vi "Streamlined FPGA--smooth window of 4.vi"() -> ()   [LabVIEW 2009]
uses:
  <vilib>/eio/EIONode/EIONode.xnode
  <vilib>/rvi/eio/nirviEIOImplementation/nirviEIOImplementation.xnode
  <vilib>/rvi/eio/common/nirviEmuTemplateMethod_noerrors.vi
  <vilib>/rvi/eio/common/nirviEmuClasses.ctl
  Instance           3 24Saved   Streamlined FPGA .vi
  Instance           4 24Saved   Streamlined FPGA .vi
  Instance           5 24Saved   Streamlined FPGA .vi
  Instance           2 24Saved   Streamlined FPGA .vi
  <vilib>/rvi/DataTransferAndStorage/Container/XNode/niFpgaContainer.xnode
  <vilib>/rvi/interface/RandomDataEmulation/niFpgaRandomDataHandleErrors.vi
  <vilib>/rvi/interface/RandomDataEmulation/nirviRandomDataFPGAFIFO.vi
  <vilib>/rvi/DataTransferAndStorage/Container/Common/niFpgaContainerMethod.ctl
  <vilib>/rvi/DataTransferAndStorage/Container/Common/niFpgaTransferTypeControl.ctl
panel:
  in  "smooth":bool
  out ">= x":bool
  out ">= y":bool
  out "xmax":i32
  out "xval":i32
  out "xmin":i32
  out ">=":bool
  in  "Rec2 Ymin":i32
  in  "Rec2 Xmin":i32
  in  "Rec1 Ymin":i32
  in  "Rec1 Xmin":i32
  in  "Rec2 Ymax":i32
  in  "Rec1 Ymax":i32
  in  "Rec2 Xmax":i32
  in  "Rec1 Xmax":i32
  out "sort!":bool
  in  "Maximum Width":i16
  in  "Maximum Height":i16
  in  "trigger on all":bool
  out "sort pulse":i16
  in  "Baselines":i16[](array[numeric])=[0, 0, 0, 0]
  in  "Sb":i8(ring)=1 items=["PMT1", "PMT2", "PMT3", "PMT4"]
  in  "Sa":i8(ring) items=["PMT1", "PMT2", "PMT3", "PMT4"]
  in  "Sort Case":i8(ring)=1 items=["FP", "Magnitude"]
  out "Full 2":bool
  in  "sort?":bool
  out "Drop counter":u32
  out "sort counter":u32
  in  "PMT to detect drops on":u8
  in  "Minimum Height":i16
  in  "Minimum Width":i16
  in  "Ticks between acquires (Ticks)":u32=200
  in  "Gain 1":i16(slide) scale=-32767.0..32767.0
  in  "Gain 2":i16(slide) scale=-32767.0..32767.0
  in  "Gain 3":i16(slide) scale=-32767.0..32767.0
  in  "Gain 4":i16(slide) scale=-32767.0..32767.0
  in  "amplitude":i16
  in  "1/Frequency \n(ticks)":u32
  in  "Burst \nCycles":i32
  in  "delay [us]":u32=20 min=1 max=8000
  # "Acquisition and Detection"
  # "FP and Sorting Parameters"
  # "Sorting Pulse\nGenerator"
  # "Events"
  # "PMT Controls"
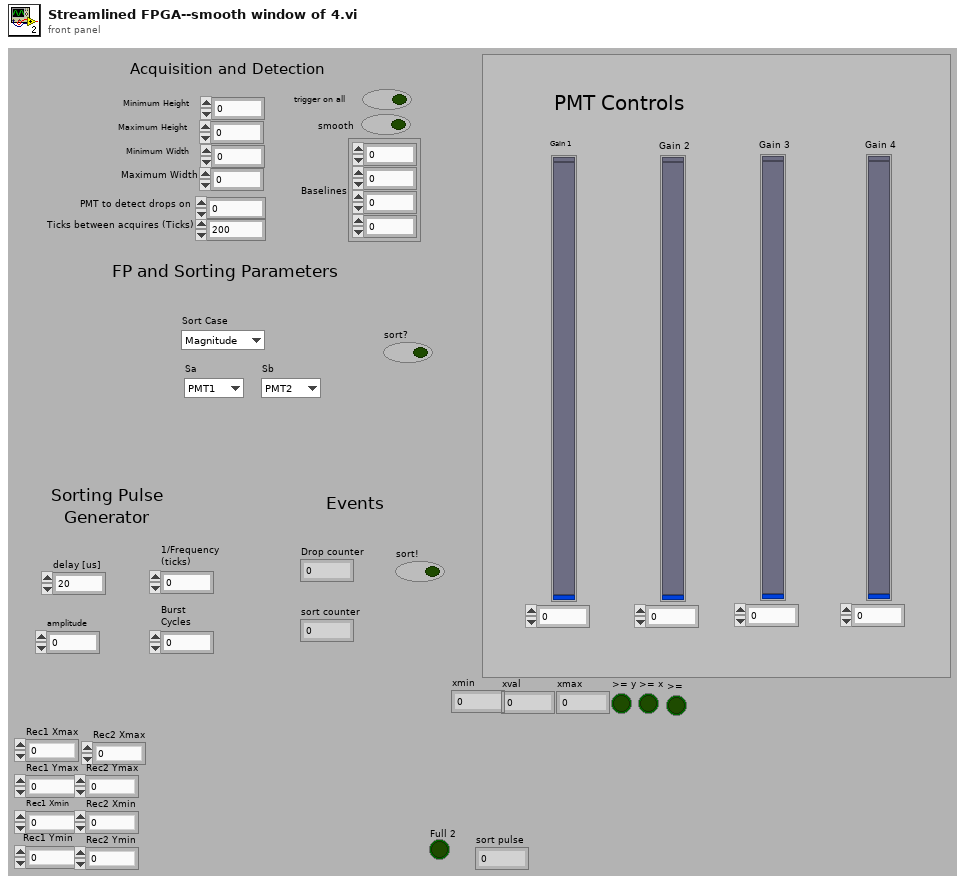
[diagram p1: front panel]
types:
  T1 = typedef "nirviEmuClasses.ctl" = enum16{"IO Read", "IO Write", "Method", "Property Read", "Property Write"}
  T2 = typedef "niFpgaContainerMethod.ctl" = enum16{"Write", "Read", "Clear", "Get Number of Elements to Write", "Get Number of Elements to Read", "Enable", "Disable", "Flush and Disable", "Get Stream State"}
  T3 = typedef "niFpgaTransferTypeControl.ctl" = enum16{"Target-Scoped", "Host to Target - DMA", "Target to Host - DMA", "Peer to Peer Reader", "Peer to Peer Writer", "Bidirectional"}
  T4 = cluster{"Rec1 Xmax":i32, "Rec1 Ymax":i32, "Rec1 Xmin":i32, "Rec1 Ymin":i32, "Rec2 Xmax":i32, "Rec2 Ymax":i32, "Rec2 Xmin":i32, "Rec2 Ymin":i32}
  T5 = cluster{bool, "max":i16[], "sum":i32[], "time inside":i32, "time outside":i32, "timeoutside-1":i32}
  T6 = cluster{"maxes":i16[], "sums":i32[], "time inside":i32, "time outside":i32}
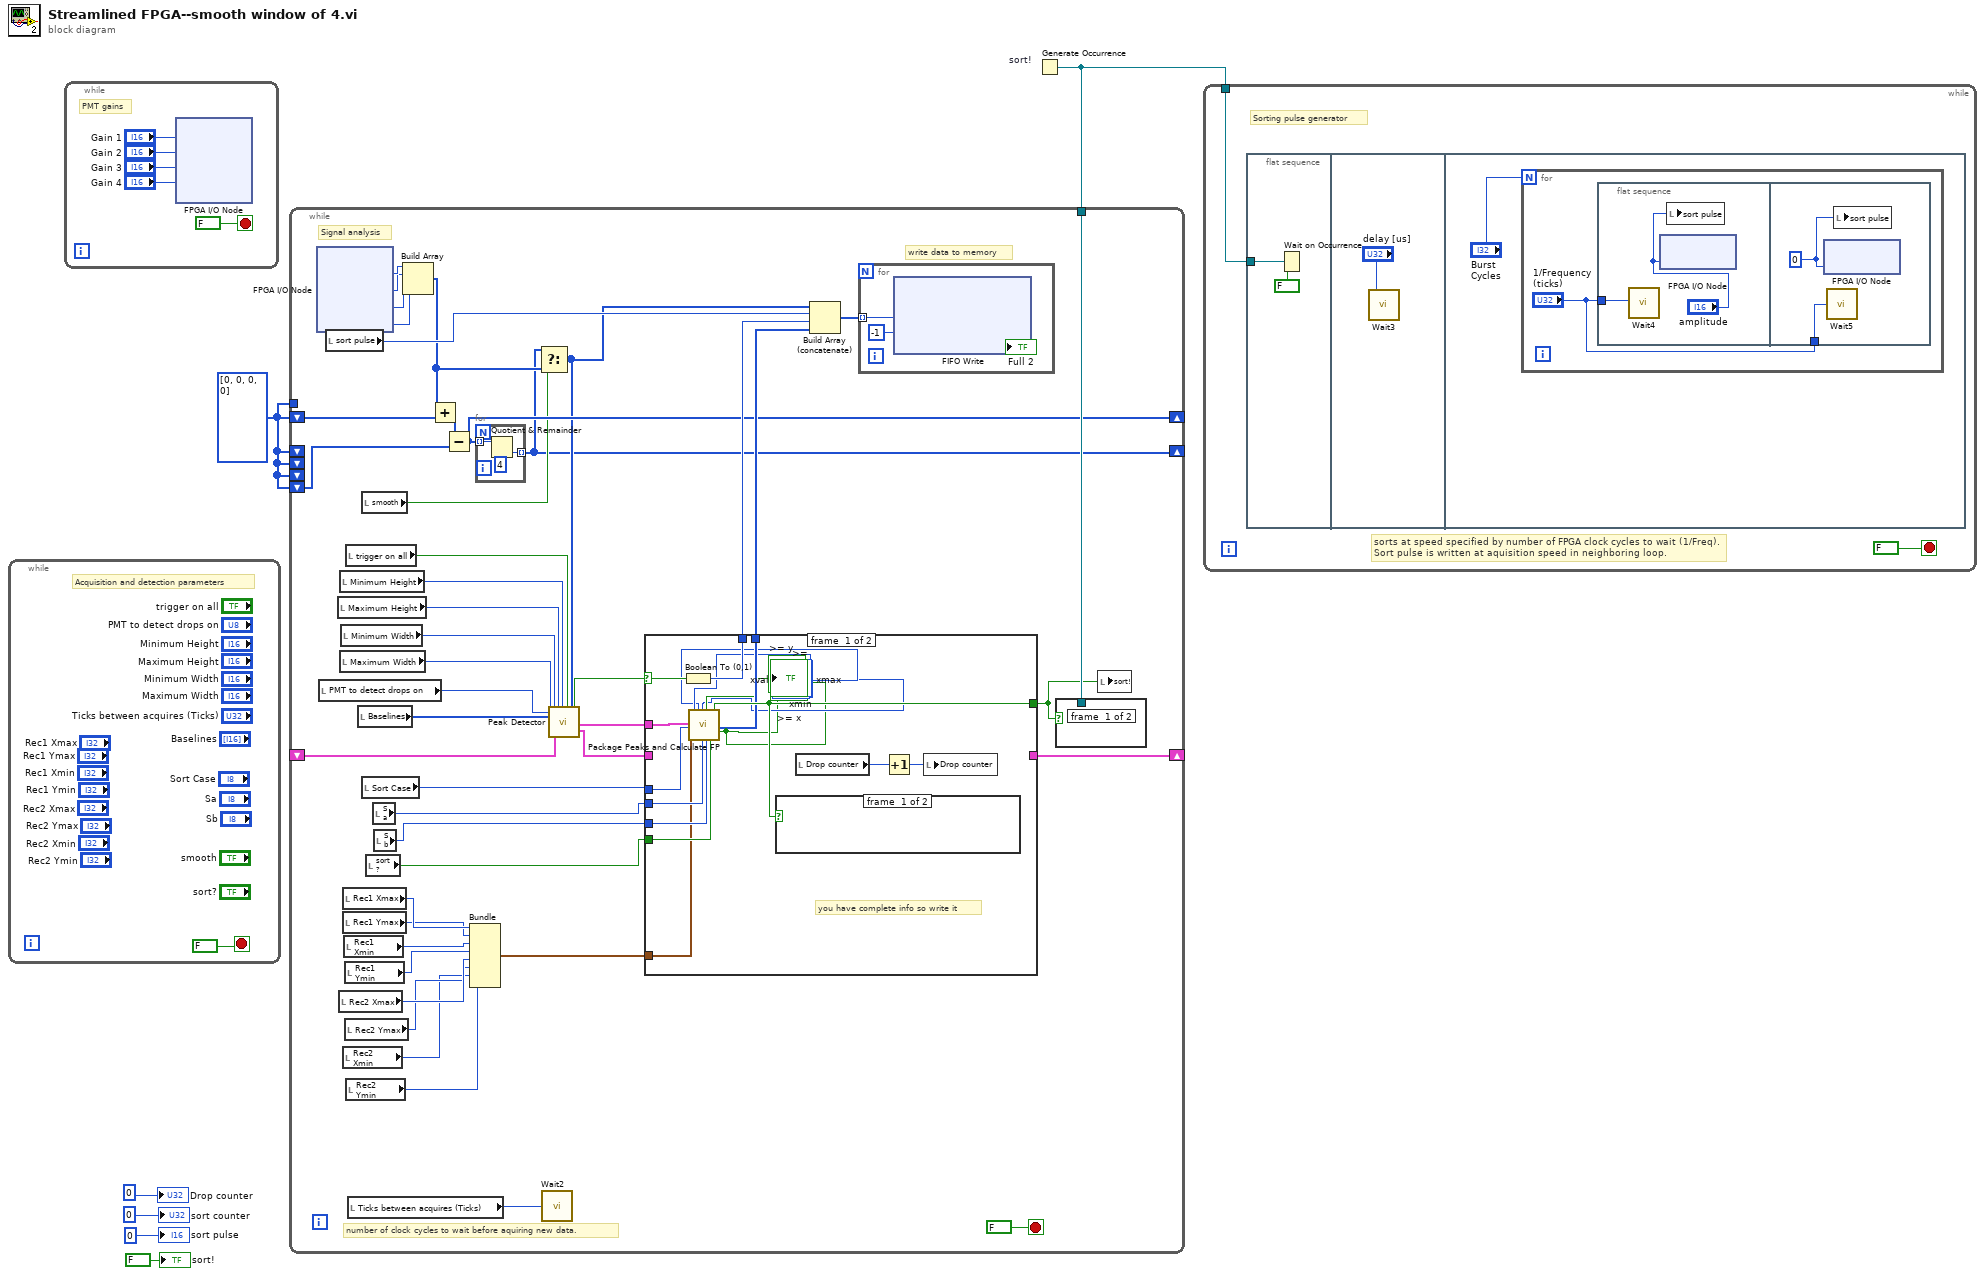
[diagram p0: block diagram]
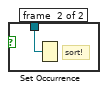
[diagram p2: hidden frame]
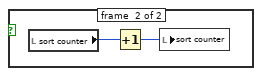
[diagram p3: hidden frame]
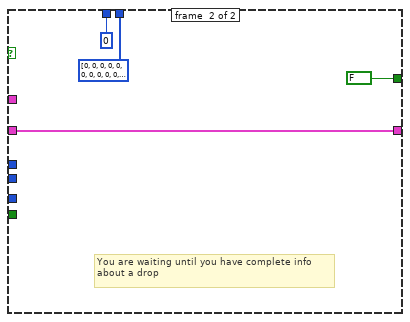
[diagram p4: hidden frame]
diagram:
  w1 = i32[] [0, 0, 0, 0] ("appended array")
  n1 = while {
    stop <- FALSE stop-if-true
    # "Acquisition and detection parameters"
  }
  n2 = while {
    stop <- FALSE stop-if-true
    # "PMT gains"
    n3 = xnode "FPGA I/O Node"("AO0"="Gain 1", "AO1"="Gain 2", "AO2"="Gain 3", "AO3"="Gain 4") -> ()  [unwired: 4 in, 4 out]
  }
  n4 = Generate Occurrence "sort!"() -> (w6:refnum<k4>)
  n5 = while {
    shift-right: [w100] -> _
    shift-left: _ -> [w87]
    tunnel: w6 -> [w85]
    shift-right: [w63] -> _
    shift-left: w1 -> [w64]
    shift-right: [w57] -> _
    shift-left: w1 -> [_]
    shift-left: w1 -> [_]
    shift-left: w1 -> [_]
    shift-left: w1 -> [w62]
    tunnel: w1 -> [_]
    stop <- FALSE stop-if-true
    # "number of clock cycles to wait before aquiring new data."
    # "Signal analysis"
    # "write data to memory"
    n6 = xnode "FPGA I/O Node"() -> ("AI0"=w99:i16, "AI1"=w98:i16, "AI2"=w97:i16, "AI3"=w96:i16)  [unwired: 4 in, 4 out]
    n7 = local read "PMT to detect drops on"() -> (w77:u8)
    n8 = local read "sort pulse"() -> (w84:i16)
    n9 = local read "Maximum Height"() -> (w80:i16)
    n10 = local read "Rec2 Xmax"() -> (w69:i32)
    n11 = local read "Minimum Height"() -> (w81:i16)
    n12 = local read "Maximum Width"() -> (w78:i16)
    n13 = local read "Minimum Width"() -> (w79:i16)
    n14 = local read "Rec1 Xmax"() -> (w73:i32)
    n15 = local read "Rec1 Ymax"() -> (w72:i32)
    n16 = local read "Rec2 Xmin"() -> (w67:i32)
    n17 = local read "Rec1 Xmin"() -> (w71:i32)
    n18 = local read "Rec1 Ymin"() -> (w70:i32)
    n19 = local read "Rec2 Ymax"() -> (w68:i32)
    n20 = local read "trigger on all"() -> (w86:bool)
    n21 = local read "Rec2 Ymin"() -> (w66:i32)
    n22 = local read "Ticks between acquires (Ticks)"() -> (w95:u32)
    n23 = local read "Baselines"() -> (w76:i16[])
    n24 = local read "smooth"() -> (w58:bool)
    n25 = local read "Sort Case"() -> (w94:i8)
    n26 = local read "sort?"() -> (w91:bool)
    n27 = local read "Sa"() -> (w93:i8)
    n28 = local read "Sb"() -> (w92:i8)
    n29 = Build Array(w99, w98, w97, w96) -> (w60:i16[])
    n30 = Add(x=w60, y=w64) -> (x+y=w61:i32[])
    n31 = Subtract(x=w61, y=w62) -> (x-y=w63:i32[])
    n32 = Bundle("Rec1 Xmax"=w73, "Rec1 Ymax"=w72, "Rec1 Xmin"=w71, "Rec1 Ymin"=w70, "Rec2 Xmax"=w69, "Rec2 Ymax"=w68, "Rec2 Xmin"=w67, "Rec2 Ymin"=w66) -> (w65:T4)  [unwired: 1 in]
    n33 = for {
      tunnel: [w103] -> w57 mode=indexing
      tunnel: w63 -> [w102] mode=indexing
      n34 = Quotient & Remainder(x=w102, y=4 ("AI3")) -> (floor(x/y)=w103:i32)  [unwired: 1 out]
    }
    n35 = Select(t=w57, s=w58, f=w60) -> (s? t:f=w59:i32[])
    n36 = call "Wait2"("Count(Ticks)"=w95) -> ()  [unwired: 1 out]
    n37 = call "Peak Detector.vi"("Maximum Width"=w78, "PMT to trigger on (0,1,2,3)"=w77, "Baselines"=w76, "Minimum Width"=w79, "shifts in"=w87, "Maximum Height"=w80, "Minimum Height"=w81, "trigger on all"=w86, "s1,s2,s3,s4"=w59) -> ("peak complete?"=w90:bool, "shifts out"=w88:T5, "peaks data"=w89:T6)  [unwired: 16 in]
    n38 = case shown="True" w90 {
      selector: w90 -> [w220 _]
      tunnel: [_ w231] -> w100
      tunnel: [w218 FALSE ("sort!")] -> w75
      tunnel: w94 -> [w216 _]
      tunnel: w93 -> [w224 _]
      tunnel: w92 -> [w223 _]
      tunnel: w91 -> [w222 _]
      tunnel: w88 -> [_ w231]
      tunnel: w89 -> [w221 _]
      tunnel: [w219 i16 0] -> w82
      tunnel: [w217 i32[] [0, 0, 0, 0, 0, 0, 0, 0, 0, 0, 0, 0] ("M1,M2,M3,M4,S1,S2,S3,S4,Tin,Tout,FP")] -> w74
      tunnel: w65 -> [w215 _]
      frame #0 {
        # "you have complete info so write it"
        n39 = Boolean To (0,1)(Boolean=w220) -> (0, 1=w219:i16)
        n40 = call "Package Peaks and Calculate FP.vi"("peaks data"=w221, "Sort Case"=w216, "Rectangle Positions"=w215, "Sa"=w224, "Sb"=w223, "sort?"=w222) -> ("xmin"=→"xmin":i32, "xval"=→"xval":i32, "xmax"=→"xmax":i32, ">="=→">=":bool, "sort!"=w218:bool, "M1,M2,M3,M4,S1,S2,S3,S4,Tin,Tout,FP,Sort?"=w217:i32[], ">= y"=→">= y" →">= x":bool)  [unwired: 14 in, 1 out]
        n41 = case shown="True" w218 {
          frame #0 {
          }
          frame #1 {
            n42 = local read "sort counter"() -> (w228:u32)
            n43 = Increment(x=w228) -> (x+1=w227:u32)
            n44 = local write "sort counter"(w227) -> ()
          }
        }
        n45 = local read "Drop counter"() -> (w226:u32)
        n46 = Increment(x=w226) -> (x+1=w225:u32)
        n47 = local write "Drop counter"(w225) -> ()
      }
      frame #1 {
        # "You are waiting until you have complete info about a drop"
      }
    }
    n48 = Build Array (concatenate)(w59, w84, w82, w74) -> (w83:i32[])
    n49 = for {
      tunnel: w83 -> [w108] mode=indexing
      n50 = xnode ("FIFO Write")("Element"=w108, "Timeout"=-1) -> ("Timed Out?"=→"Full 2":bool)  [unwired: 1 in, 1 out]
    }
    n51 = case shown="True" w75 {
      tunnel: w85 -> [_ w105]
      frame #0 {
      }
      frame #1 {
        # "sort!"
        n52 = Set Occurrence(w105) -> ()
      }
    }
    n53 = local write "sort!"(w75) -> ()
  }
  n54 = while {
    tunnel: w6 -> [w233]
    stop <- FALSE stop-if-true
    # "sorts at speed specified by number of FPGA clock cycles to wait (1/Freq).\nSort pulse is written at aquisition speed in neighboring loop."
    # "Sorting pulse generator"
    n55 = flat-sequence {
      tunnel: w233 -> [w235]
      frame #0 {
        n56 = Wait on Occurrence(1:FALSE ("ignore previous (T)"), 2:w235) -> ()  [unwired: 1 in, 1 out]
      }
      frame #1 {
        n57 = call "Wait3"("Count(uSec)"="delay [us]") -> ()  [unwired: 1 out]
      }
      frame #2 {
        n58 = for {
          N: "Burst \nCycles" -> [_]
          n59 = flat-sequence {
            tunnel: "1/Frequency \n(ticks)" -> [w241]
            tunnel: "1/Frequency \n(ticks)" -> [w254]
            frame #0 {
              n60 = call "Wait4"("Count(Ticks)"=w241) -> ()  [unwired: 1 out]
              n61 = xnode "FPGA I/O Node"("AO4"="amplitude") -> ()  [unwired: 1 in, 1 out]
              n62 = local write "sort pulse"("amplitude") -> ()
            }
            frame #1 {
              w253 = i16 0 ("sort pulse")
              n63 = xnode "FPGA I/O Node"("AO4"=w253) -> ()  [unwired: 1 in, 1 out]
              n64 = call "Wait5"("Count(Ticks)"=w254) -> ()  [unwired: 1 out]
              n65 = local write "sort pulse"(w253) -> ()
            }
          }
        }
      }
    }
  }
  "sort counter" <- u32 0 ("event counter")
  "Drop counter" <- u32 0 ("Drop counter")
  "sort pulse" <- i16 0 ("event counter")
  "sort!" <- FALSE ("sort!")
